vi "Read Data.vi"(8 "error in (no error)":errorcluster, 11 "String Data in":refnum<class "String Data.lvclass">) -> (0 "error out":errorcluster, 2 "Data":string, 3 "String Data out":refnum<class "String Data.lvclass">)   [LabVIEW 2016, in "String Data.lvclass"]
uses:
  String Data.lvclass
  String Data.lvclass/String Data.ctl
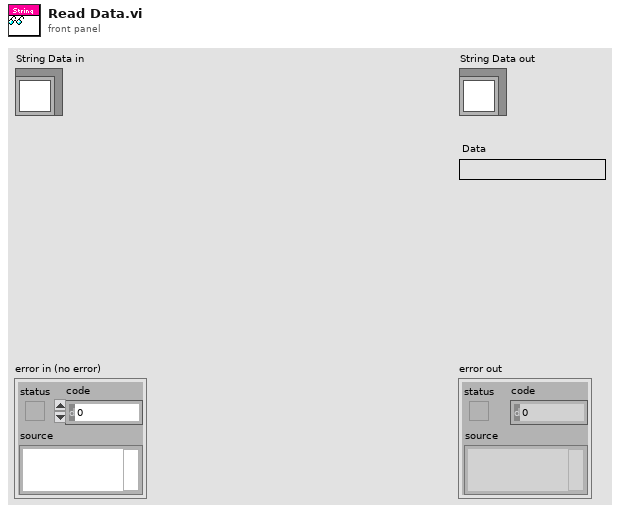
[diagram p1: front panel]
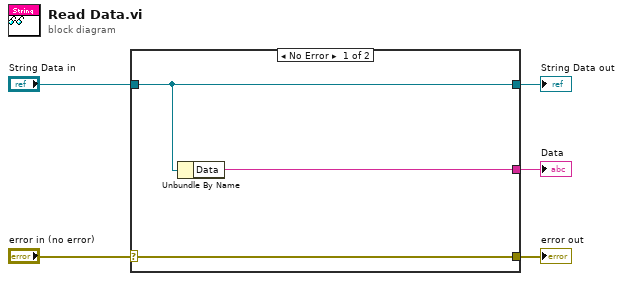
[diagram p0: block diagram]
diagram:
  n1 = case shown="No Error" "error in (no error)" {
    selector: "error in (no error)" -> [w8 w9]
    tunnel: [w8 w9] -> w4
    tunnel: [w7 w10] -> w2
    tunnel: "String Data in" -> [w7 w10]
    tunnel: [w6 _] -> w1
    frame No Error {
      n2 = Unbundle By Name(w7) -> ("Data"=w6:string)
    }
    frame Error {
    }
  }
  "error out" <- w4
  "String Data out" <- w2
  "Data" <- w1
